vi "sweep_fields.vi"(6 "Axis":string, 8 "Queue":string[][](table)=[["Formula", "Start", "Finish", "Points", "Time"], ["t", "3", "5", "100", "600"], ["", "", "", "", ""]], 9 "Max Sweep Rates":dbl[][](array[numeric]), 10 "Loop":bool, 11 "VISA In":refnum<visa-resource-name>) -> (3 "VISA Out":refnum<visa-resource-name>)   [LabVIEW 2016]
uses:
  <vilib>/gmath/NI_Gmath.lvlib
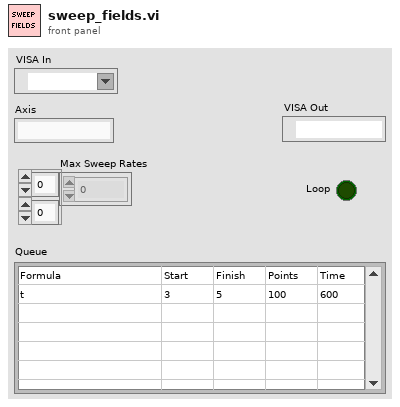
[diagram p1: front panel]
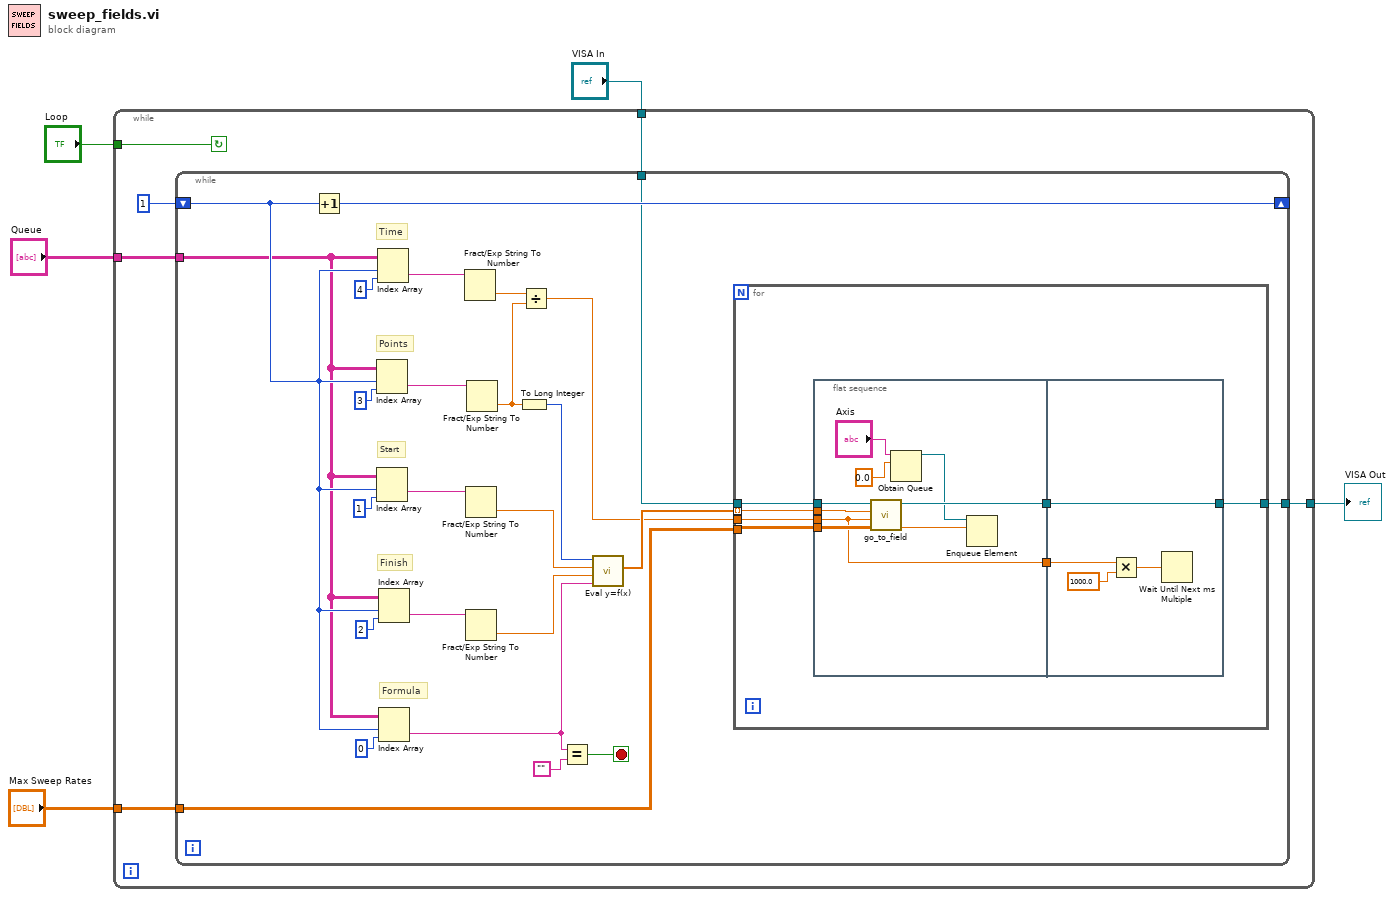
[diagram p0: block diagram]
diagram:
  n1 = while {
    tunnel: "Queue" -> [w10]
    tunnel: "Max Sweep Rates" -> [w9]
    tunnel: [w8] -> w3
    tunnel: "VISA In" -> [w7]
    tunnel: "Loop" -> [w6]
    stop <- w6 continue-if-true
    n2 = while {
      shift-right: [w20] -> _
      shift-left: 1 ("disabled index (col)") -> [w18]
      tunnel: w10 -> [w17]
      tunnel: [w16] -> w8
      tunnel: w9 -> [w13]
      tunnel: w7 -> [w12]
      stop <- w19 stop-if-true
      # "Time"
      # "Points"
      # "Formula"
      # "Finish"
      # "Start"
      n3 = Increment(x=w18) -> (x+1=w20:i32)
      n4 = Index Array(array=w17, index (row)=w18, index (col)=3 ("disabled index (col)")) -> (element=w30:string)
      n5 = Index Array(array=w17, index (row)=w18, index (col)=1) -> (element=w33:string)
      n6 = Index Array(array=w17, index (row)=w18, index (col)=4) -> (element=w26:string)
      n7 = Index Array(array=w17, index (row)=w18, index (col)=2) -> (element=w32:string)
      n8 = Index Array(array=w17, index (row)=w18, index (col)=0) -> (element=w22:string)
      n9 = Fract/Exp String To Number(string=w26) -> (number=w25:dbl)  [unwired: 3 in, 1 out]
      n10 = Fract/Exp String To Number(string=w33) -> (number=w29:dbl)  [unwired: 3 in, 1 out]
      n11 = Fract/Exp String To Number(string=w32) -> (number=w28:dbl)  [unwired: 3 in, 1 out]
      n12 = Fract/Exp String To Number(string=w30) -> (number=w24:dbl)  [unwired: 3 in, 1 out]
      n13 = To Long Integer(number=w24) -> (32bit integer=w23:i32)
      n14 = Divide(x=w25, y=w24) -> (x/y=w14:dbl)
      n15 = Equal?(x=w22, y="") -> (x = y?=w19:bool)
      n16 = call <vilib>:"Eval y=f(x).vi"("formula"=w22, "end"=w28, "start"=w29, "number of points"=w23) -> ("Y Values"=w15:dbl[])  [unwired: 3 out]
      n17 = for {
        tunnel: w15 -> [w43] mode=indexing
        tunnel: w12 -> [w42]
        tunnel: w14 -> [w41]
        tunnel: w13 -> [w40]
        tunnel: [w37] -> w16
        n18 = flat-sequence {
          tunnel: w43 -> [w52]
          tunnel: w42 -> [w51]
          tunnel: w41 -> [w49]
          tunnel: w40 -> [w50]
          tunnel: [w49] -> w39
          tunnel: [w48] -> w38
          tunnel: w39 -> [w54]
          tunnel: [w53] -> w37
          tunnel: w38 -> [w53]
          frame #0 {
            n19 = call "go_to_field.vi"("Max Rates"=w50, "Timestep"=w49, "Sweep To"=w52, "VISA In"=w51) -> ("B-Field"=w47:dbl, "VISA Out"=w48:refnum<visa-resource-name>)  [unwired: 6 in]
            n20 = Obtain Queue(name (unnamed)="Axis", element data type=0.0 ("y")) -> (queue out=w46:refnum<queue>)  [unwired: 3 in, 2 out]
            n21 = Enqueue Element(queue=w46, element=w47) -> ()  [unwired: 2 in, 3 out]
          }
          frame #1 {
            n22 = Multiply(x=w54, y=1000.0) -> (x*y=w55:dbl)
            n23 = Wait Until Next ms Multiple(millisecond multiple=w55) -> ()  [unwired: 1 out]
          }
        }
      }
    }
  }
  "VISA Out" <- w3
